vi "GetVolume.vi"(8 "error in (no error)":errorcluster, 11 "SeriesURL":string) -> (0 "error out":errorcluster, 3 "Volume":i32)   [LabVIEW 2022 SP3]
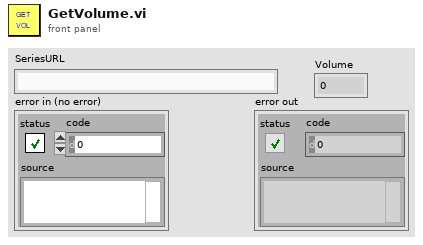
[diagram p1: front panel]
types:
  T1 = typedef "Series.ctl" = cluster{"URL":string, "Volume":i32, "StartYear":i32, "EndYear":i32, "Active?":bool}
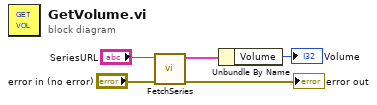
[diagram p0: block diagram]
diagram:
  n1 = call "FetchSeries.vi"("error in (no error)"="error in (no error)", "SeriesURL"="SeriesURL") -> ("error out"=→"error out":errorcluster, "Series"=w3:T1)  [unwired: 8 in]
  n2 = Unbundle By Name(w3) -> ("Volume"=→"Volume":i32)
